vi "NET Tester.vi"() -> ()   [LabVIEW 2023]
uses:
  NationalInstruments.UI.Styles3D
  System.Windows.Forms
  System.Drawing
  NationalInstruments.UI
  NationalInstruments.UI.WindowsForms
panel:
  out "Style ID":u32
  out "ToString 3":string
  out "value__":i32
  in  "File Path":path
  out "ContainsImage":bool
  out "ToString 2":string
  out "ToString":string
  in  "Button 2":bool
  in  "Button":bool
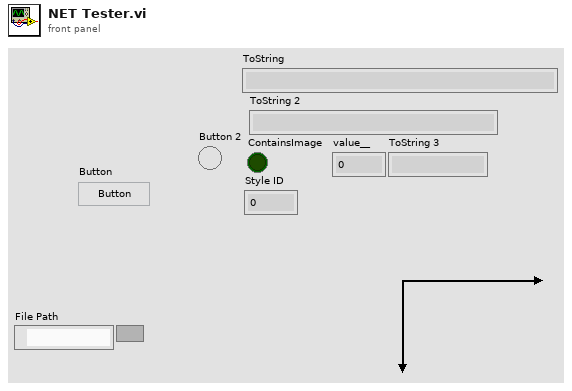
[diagram p1: front panel]
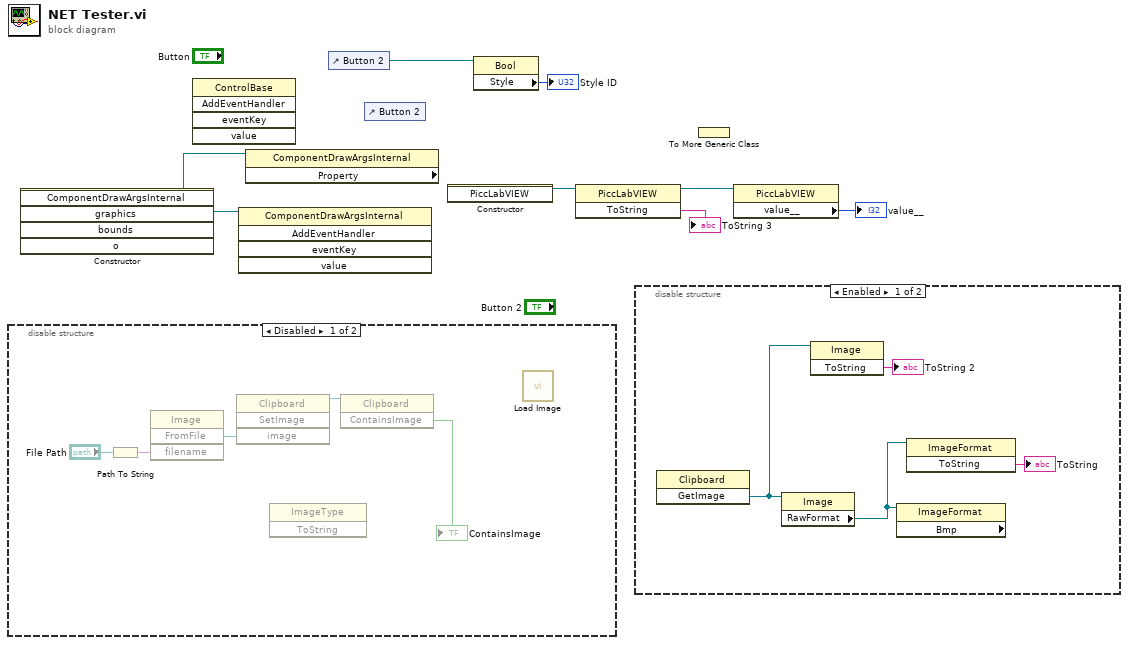
[diagram p0: block diagram]
diagram:
  n1 = disable-structure shown="Disabled" {
    frame Disabled {
      n2 = Path To String(path="File Path") -> (string=w10:string)
      n3 = invoke class="Image" method="FromFile"("filename"=w10) -> ("FromFile"=w9:refnum<k24>)  [unwired: 3 in, 3 out]
      n4 = invoke class="Clipboard" method="SetImage"("image"=w9) -> (reference out=w8:refnum<k24>)  [unwired: 3 in, 3 out]
      n5 = invoke class="ImageType" method="ToString"() -> ()  [unwired: 3 in, 3 out]
      n6 = invoke class="Clipboard" method="ContainsImage"(reference=w8) -> ("ContainsImage"=→"ContainsImage":bool)  [unwired: 2 in, 2 out]
      n7 = call <userlib>:"Load Image.vi"() -> ()  [unwired: 9 in, 3 out]
    }
    frame Enabled {
    }
  }
  n8 = constructor class="ComponentDrawArgsInternal"() -> (reference out=w1:refnum<k24>)  [unwired: 6 in, 5 out]
  n9 = invoke class="ControlBase" method="AddEventHandler"() -> ()  [unwired: 5 in, 5 out]
  n10 = invoke class="ComponentDrawArgsInternal" method="AddEventHandler"(reference=w1) -> ()  [unwired: 4 in, 5 out]
  n11 = property class="ComponentDrawArgsInternal" props=[](reference=w1) -> ()  [unwired: 1 in, 3 out]
  n12 = control-ref of="Button 2"() -> (w3:refnum<vi>)
  n13 = control-ref of="Button 2"() -> ()  [unwired: 1 out]
  n14 = constructor class="PiccLabVIEW"() -> (reference out=w6:refnum<k24>)  [unwired: 3 in, 2 out]
  n15 = property class="Bool"(reference=w3) -> ("Style"=→"Style ID":u32)  [unwired: 1 in, 2 out]
  n16 = invoke class="PiccLabVIEW" method="ToString"(reference=w6) -> (reference out=w5:refnum<k24>, "ToString"=→"ToString 3":string)  [unwired: 2 in, 1 out]
  n17 = disable-structure shown="Enabled" {
    frame Enabled {
      n18 = invoke class="Clipboard" method="GetImage"() -> ("GetImage"=w14:refnum<k24>)  [unwired: 3 in, 2 out]
      n19 = property class="Image"(reference=w14) -> ("RawFormat"=w13:refnum<k24>)  [unwired: 1 in, 2 out]
      n20 = invoke class="Image" method="ToString"(reference=w14) -> ("ToString"=→"ToString 2":string)  [unwired: 2 in, 2 out]
      n21 = property class="ImageFormat" props=["Bmp"](reference=w13) -> ()  [unwired: 1 in, 3 out]
      n22 = invoke class="ImageFormat" method="ToString"(reference=w13) -> ("ToString"=→"ToString":string)  [unwired: 2 in, 2 out]
    }
    frame Disabled {
    }
  }
  n23 = To More Generic Class() -> ()  [unwired: 2 in, 1 out]
  n24 = property class="PiccLabVIEW"(reference=w5) -> ("value__"=→"value__":i32)  [unwired: 1 in, 2 out]
